vi "18.3.1 Location-Inspection.vi"() -> ()   [LabVIEW 2017]
doc: "This example illustrates the use of the horizontal clamp tool. You can draw a region of inspection that contains at least two edges in the image. The VI measures the distance between the first and last edges."
uses:
  <vilib>/vision/NI_Vision_Development_Module.lvlib
panel:
  out "Total Located:":i32
  out "Pass?":bool
  in  "Stop":bool
  in  "Delay(s)":dbl(slide)=1.0285714285714285 scale=0.0..3.0
  out "UUT":T1(plugin-control)
  out "TMP":T1(plugin-control)
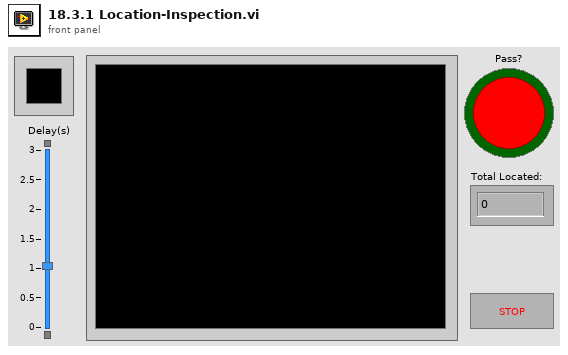
[diagram p1: front panel]
types:
  T1 = typedef "IMAQ Image.ctl" = refnum<image>
  T2 = typedef "Image Type" = u32
  T3 = cluster{"Position":cluster{"x":sgl, "y":sgl}, "Angle":sgl, "Scale":sgl, "Score":sgl, "Bounding Box":cluster{"x":sgl, "y":sgl}[]}[]
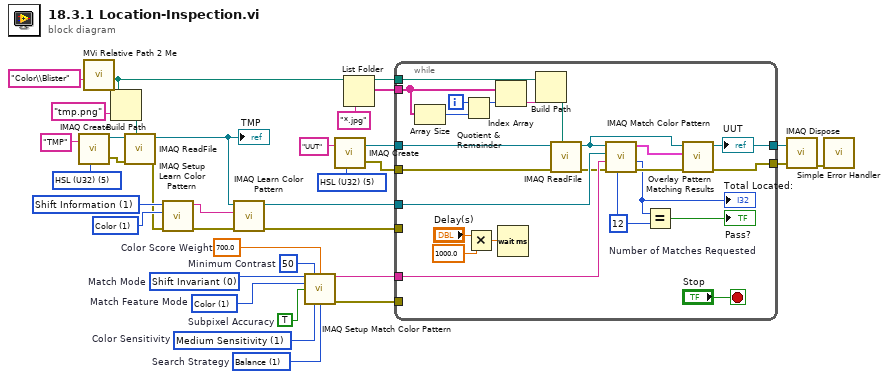
[diagram p0: block diagram]
diagram:
  w13 = TRUE  # Subpixel Accuracy
  w11 = u32 1 items=["Color and Shape", "Color", "Shape"]  # Match Feature Mode
  w7 = u32 1 items=["Conservative", "Balance", "Aggressive", "Very Aggressive"]  # Search Strategy
  w10 = 50  # Minimum Contrast
  w9 = sgl 700.0  # Color Score Weight
  w8 = u32 1 items=["Low Sensitivity", "Medium Sensitivity", "High Sensitivity"]  # Color Sensitivity
  w12 = u32 0 items=["Shift Invariant", "Rotation Invariant"]  # Match Mode
  w17 = u32 1 items=["Color and Shape", "Color", "Shape "] ("Feature Mode")
  w16 = u32 1 items=["All", "Shift Information", "Rotation Information"] ("Learn Mode")
  w30 = T2 5 items=["Grayscale (U8)", "Grayscale (I16)", "Grayscale (SGL)", "Complex (CSG)", "RGB (U32)", "HSL (U32)", "RGB (U64)", "Grayscale (U16)"] ("Image Type")
  w32 = T2 5 items=["Grayscale (U8)", "Grayscale (I16)", "Grayscale (SGL)", "Complex (CSG)", "RGB (U32)", "HSL (U32)", "RGB (U64)", "Grayscale (U16)"] ("Image Type")
  n1 = call "IMAQ Create"("Image Name"="TMP", "Image Type"=w32) -> ("New Image"=w31:T1, "error out"=w26:errorcluster)  [unwired: 3 in]
  n2 = call "MVi Relative Path 2 Me.vi"("Relative Path"="Color\\Blister" ("name or relative path")) -> ("Appended Dir"=w21:path)  [unwired: 5 in, 1 out]
  n3 = Build Path(base path=w21, name or relative path="tmp.png") -> (appended path=w24:path)
  n4 = call "IMAQ ReadFile"("File Path"=w24, "error in (no error)"=w26, "Image"=w31) -> ("error out"=w3:errorcluster, "Image Out"=w4:T1)  [unwired: 4 in, 3 out]
  "TMP" <- w4
  n5 = call "IMAQ Setup Learn Color Pattern"("error in (no error)"=w3, "Feature Mode"=w17, "Learn Mode"=w16) -> ("error out"=w15:errorcluster, "Learn Color Pattern Setup Data"=w14:string)  [unwired: 7 in]
  n6 = call "IMAQ Learn Color Pattern"("error in (no error)"=w15, "Learn Color Pattern Setup Data"=w14, "Image"=w4) -> ("error out"=w6:errorcluster, "Template Image Out"=w5:T1)  [unwired: 7 in]
  n7 = call "IMAQ Setup Match Color Pattern"("Match Mode"=w12, "Minimum Contrast"=w10, "Color Score Weight"=w9, "Match Feature Mode"=w11, "Subpixel Accuracy"=w13, "Color Sensitivity"=w8, "Search Strategy"=w7) -> ("Match Color Pattern Setup Data"=w1:string, "error out"=w2:errorcluster)  [unwired: 7 in]
  n8 = call "IMAQ Create"("Image Name"="UUT", "Image Type"=w30) -> ("New Image"=w28:T1, "error out"=w27:errorcluster)  [unwired: 3 in]
  n9 = List Folder(path=w21, pattern="*.jpg") -> (path out=w19:path, filenames=w18:string[])  [unwired: 2 in, 2 out]
  n10 = while {
    tunnel: w19 -> [w58]
    tunnel: w18 -> [w51]
    tunnel: w6 -> [_]
    tunnel: w5 -> [w46]
    tunnel: w2 -> [_]
    tunnel: w1 -> [w45]
    tunnel: w28 -> [w47]
    tunnel: [w39] -> w22
    tunnel: w27 -> [w59]
    tunnel: [w41] -> w23
    i -> [w53]
    stop <- "Stop" stop-if-true
    w38 = 12  # Number of Matches Requested
    n11 = Array Size(array=w51) -> (size(s)=w52:i32)
    n12 = Quotient & Remainder(x=w53, y=w52) -> (x-y*floor(x/y)=w48:i32)  [unwired: 1 out]
    n13 = Multiply(x="Delay(s)", y=1000.0) -> (x*y=w54:dbl)
    n14 = Index Array(array=w51, index=w48) -> (element=w50:string)
    n15 = Wait (ms)(milliseconds to wait=w54) -> ()  [unwired: 1 out]
    n16 = Build Path(base path=w58, name or relative path=w50) -> (appended path=w57:path)
    n17 = call "IMAQ ReadFile"("File Path"=w57, "error in (no error)"=w59, "Image"=w47) -> ("error out"=w44:errorcluster, "Image Out"=w40:T1)  [unwired: 4 in, 3 out]
    n18 = call "IMAQ Match Color Pattern"("Number of Matches Requested"=w38, "error in (no error)"=w44, "Match Color Pattern Setup Data"=w45, "Template Image"=w46, "Image"=w40) -> ("error out"=w43:errorcluster, "Number of Matches"=w36:i32, "Matches"=w42:T3)  [unwired: 4 in]
    "Total Located:" <- w36
    n19 = Equal?(x=w36, y=w38) -> (x = y?=→"Pass?":bool)
    n20 = call "Overlay Pattern Matching Results.vi"("error in"=w43, "Matches"=w42, "Image"=w40) -> ("error out"=w41:errorcluster, "Image Out"=w39:T1)  [unwired: 7 in]
    "UUT" <- w39
  }
  n21 = call "IMAQ Dispose"("Image"=w22, "error in (no error)"=w23) -> ("error out"=w35:errorcluster)  [unwired: 4 in]
  n22 = call <vilib>:"Simple Error Handler.vi"("error in (no error)"=w35) -> ()  [unwired: 4 in, 5 out]
